vi "Add Tool.vi"(2 "Exception Values":string[](array[string]), 4 "ignored?":bool[](array[boolean]), 5 "Parameter Types":T1[](array[typedef]), 6 "Input?":bool[](array[boolean]), 7 "Parameter Names":string[](array[string]), 8 "error in (no error)":errorcluster, 9 "Description":string, 10 "Name":string, 11 "PyServer in":refnum<class "PyServer.lvclass">) -> (0 "error out":errorcluster, 3 "PyServer out":refnum<class "PyServer.lvclass">)   [LabVIEW 2025, in "Tools.lvlib" / "PyServer.lvclass"]
uses:
  PyServer.lvclass
  Datatypes.ctl
  Toolset.ctl
  PyServer.lvclass/PyServer.ctl
  Tools.lvlib
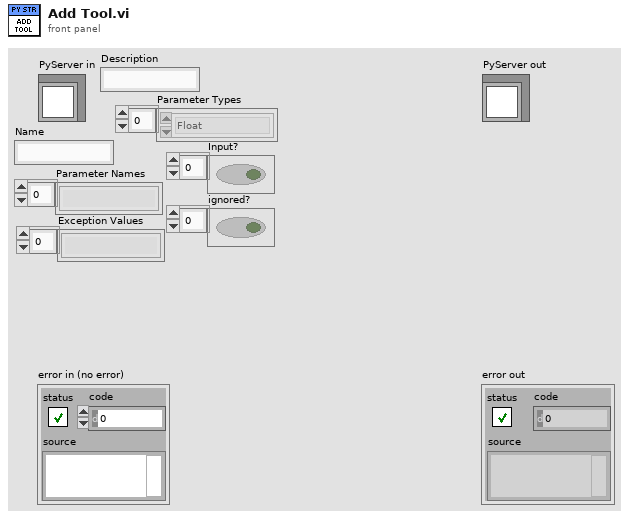
[diagram p1: front panel]
types:
  T1 = typedef "Tools.lvlib/Datatypes.ctl" = enum16{"Float", "Int", "String", "String Array", "Int Array", "Float Array", "Bool Array", "Bool", "Invalid"}
  T2 = typedef "Tools.lvlib/PyServer.lvclass/Toolset.ctl" = cluster{"Name":string, "Description":string, "Parameter Names":string[], "Parameter Types":T1[], "Input?":bool[], "ignored?":bool[], "Exception Values":string[]}
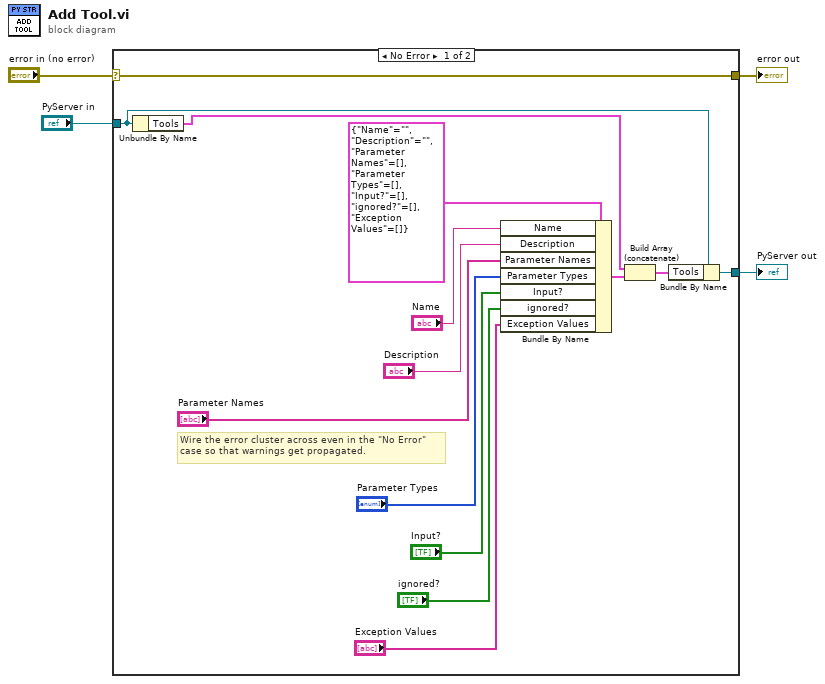
[diagram p0: block diagram]
diagram:
  n1 = case shown="No Error" "error in (no error)" {
    selector: "error in (no error)" -> [w18 w20]
    tunnel: [w18 w20] -> w3
    tunnel: [w17 w19] -> w1
    tunnel: "PyServer in" -> [w16 w19]
    frame No Error {
      # "Wire the error cluster across even in the \"No Error\"\ncase so that warnings get propagated."
      n2 = Unbundle By Name(w16) -> ("Tools"=w15:T2[])
      n3 = Bundle By Name(cluster=T2 {"Name"="", "Description"="", "Parameter Names"=[], "Parameter Types"=[], "Input?"=[], "ignored?"=[], "Exception Values"=[]} ("Tool"), "Name"="Name", "Description"="Description", "Parameter Names"="Parameter Names", "Parameter Types"="Parameter Types", "Input?"="Input?", "ignored?"="ignored?", "Exception Values"="Exception Values") -> (w13:T2)
      n4 = Build Array (concatenate)(w15, w13) -> (w14:T2[])
      n5 = Bundle By Name(cluster=w16, "Tools"=w14) -> (w17:refnum<class "PyServer.lvclass">)
    }
    frame Error {
    }
  }
  "error out" <- w3
  "PyServer out" <- w1
